vi "XIPIN_AXI_Traffic_Generator_2_0.vi"   [LabVIEW 2017]
doc: "AXI Traffic Generator genertes AXI traffic based on core programming\n------------------------------------\n<b>Need License</b> : No\n<b>Interface</b> : AXI4 AXI4-Stream"
uses:
  <vilib>/rvi/XilinxIP/XIPIN_XNode/niFpgaXIPIN.xnode
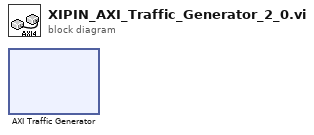
[diagram p0: block diagram]
diagram:
  n1 = xnode ("AXI Traffic Generator")() -> ()
